vi "Turn Right.vi"() -> ()   [LabVIEW 2017]
uses:
  <vilib>/Rock Robotics/SystemInterfaces/DIO/FPGA_DIOPWMChannel.ctl
  <vilib>/Rock Robotics/SystemInterfaces/DIO/FPGA_DIOChannel.ctl
  <vilib>/Rock Robotics/WPI/MotorControl/WPI_MotorControlOpen SPARK.vi
  <vilib>/Rock Robotics/WPI/Counter/WPI_CounterDigitalInputToDigitalSource.vi
panel:
  out "Distance 2":dbl
  out "Distance":dbl
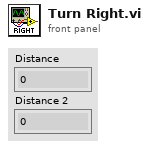
[diagram p1: front panel]
types:
  T1 = typedef "FPGA_DIOChannel.ctl" = enum8{"DIO 0", "DIO 1", "DIO 2", "DIO 3", "DIO 4", "DIO 5", "DIO 6", "DIO 7", "DIO 8", "DIO 9", "DIO MXP 0", "DIO MXP 1", "DIO MXP 2", "DIO MXP 3", "DIO MXP 4", "DIO MXP 5", "DIO MXP 6", "DIO MXP 7", "DIO MXP 8", "DIO MXP 9", "DIO MXP 10", "DIO MXP 11", "DIO MXP 12", "DIO MXP 13", "DIO MXP 14", "DIO MXP 15", "SPI Port CS1", "SPI Port CS2", "SPI Port CS3", "SPI Port MISO", "SPI Port MOSI", "Invalid"}
  T2 = typedef "FPGA_DIOPWMChannel.ctl" = enum8{"PWM 0", "PWM 1", "PWM 2", "PWM 3", "PWM 4", "PWM 5", "PWM 6", "PWM 7", "PWM 8", "PWM 9", "PWM MXP 0", "PWM MXP 1", "PWM MXP 2", "PWM MXP 3", "PWM MXP 4", "PWM MXP 5", "PWM MXP 6", "PWM MXP 7", "PWM MXP 8", "PWM MXP 9", "Invalid"}
  T3 = typedef "WPI_DigitalInputDevRef.ctl" = cluster{"DevStatus":errorcluster, "DIO Channel":T1}
  T4 = typedef "FPGA_CounterEncoderSourceConvertionLVSourceType.ctl" = cluster{"DevStatus":errorcluster, "AnalogTriggerMode?":bool, "DigitalMode":cluster{"DIO Channel":T5}, "AnalogTriggerMode":cluster{"AnalogTriggerIndex":T6, "OutputType":T7}}
  T5 = typedef "FPGA_DIODigitalSourceChannel.ctl" = enum8{"DIO 0", "DIO 1", "DIO 2", "DIO 3", "DIO 4", "DIO 5", "DIO 6", "DIO 7", "DIO 8", "DIO 9", "DIO MXP 0", "DIO MXP 1", "DIO MXP 2", "DIO MXP 3", "DIO MXP 4", "DIO MXP 5", "DIO MXP 6", "DIO MXP 7", "DIO MXP 8", "DIO MXP 9", "DIO MXP 10", "DIO MXP 11", "DIO MXP 12", "DIO MXP 13", "DIO MXP 14", "DIO MXP 15", "Disabled"}
  T6 = typedef "FPGA_AnalogTriggerIndex.ctl" = enum8{"Trig 0", "Trig 1", "Trig 2", "Trig 3", "Trig 4", "Trig 5", "Trig 6", "Trig 7", "Invalid"}
  T7 = typedef "FPGA_AnalogTriggerOutType.ctl" = enum16{"InWindow", "TriggerState", "Rising", "Falling"}
  T8 = typedef "WPI_EncoderDevRef.ctl" = cluster{"DevStatus":errorcluster, "EncoderIndex":T9, "CounterIndex":T10, "DistancePerCount":dbl, "Decoding Type":T11}
  T9 = typedef "FPGA_EncoderIdx.ctl" = enum8{"Enc 0", "Enc 1", "Enc 2", "Enc 3", "Enc 4", "Enc 5", "Enc 6", "Enc 7", "Invalid"}
  T10 = typedef "FPGA_CounterCtrSystemIndex.ctl" = enum8{"Ctr 0", "Ctr 1", "Ctr 2", "Ctr 3", "Ctr 4", "Ctr 5", "Ctr 6", "Ctr 7", "Invalid"}
  T11 = typedef "WPI_EncoderType.ctl" = enum16{"1x", "2x", "4x"}
  T12 = typedef "WPI_MotorControlDeviceRef.ctl" = cluster{"DeviceStatus":errorcluster, "Type":T13, "PWM":cluster{"PWM Channel":T2, "DeadBand":T14}, "CAN":cluster{"Device Number":u8, "SetOutput VI Ref":variant, "GetOutput VI Ref":variant, "Enable VI Ref":variant, "Disable VI Ref":variant, "Data":variant}, "Invert":bool, "DIO PWM":cluster{"PWM \"Enable\" Channel":T2, "DIOChannel":T1, "PWM Rate":dbl}}
  T13 = typedef "WPI_MotorControlType.ctl" = enum16{"PWM", "CAN", "DIO PWM"}
  T14 = typedef "WPI_PWMDeadband.ctl" = cluster{"Name":string, "maxPositivePwm":i32, "minPositivePwm":i32, "centerPwm":i32, "maxNegativePwm":i32, "minNegativePwm":i32, "angularRange":u16}
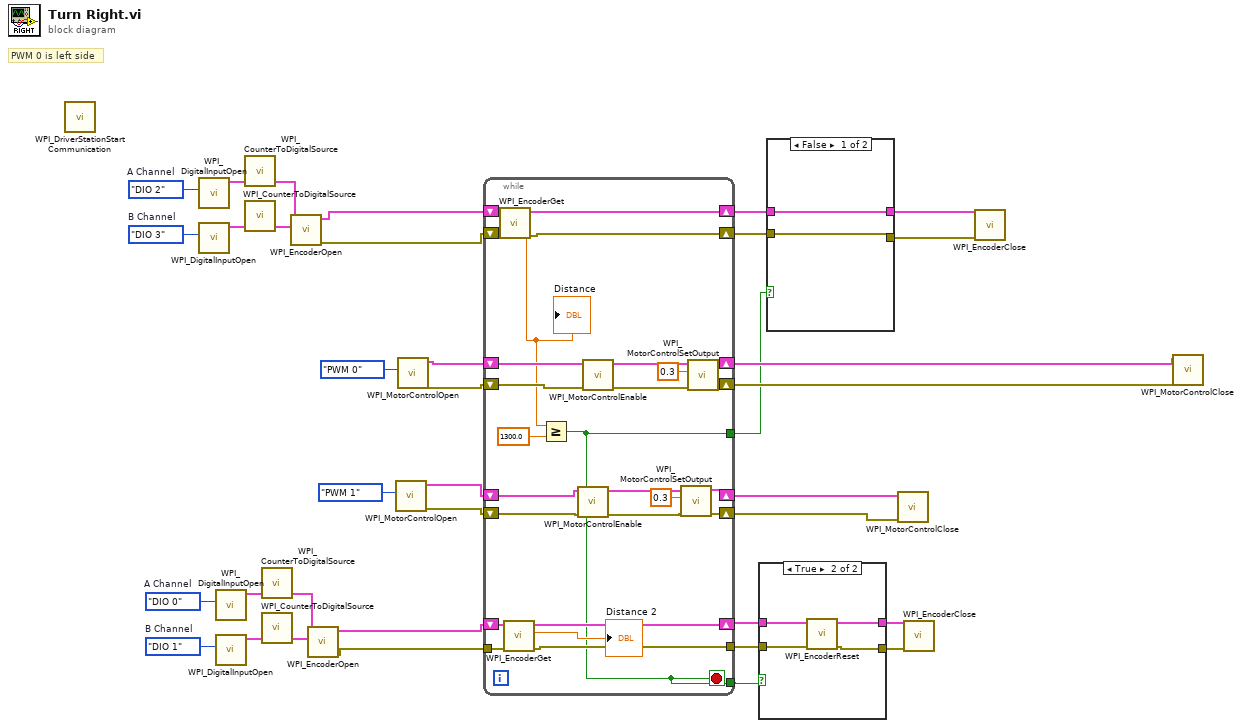
[diagram p0: block diagram]
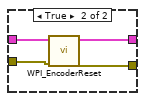
[diagram p3: hidden frame]
diagram:
  w13 = FPGA_DIOChannel."DIO 1"  # B Channel
  w14 = FPGA_DIOChannel."DIO 0"  # A Channel
  w33 = FPGA_DIOChannel."DIO 3"  # B Channel
  w32 = FPGA_DIOChannel."DIO 2"  # A Channel
  # "PWM 0 is left side"
  n1 = call <vilib>:"WPI_DriverStationStart Communication.vi"() -> ()  [unwired: 12 in]
  n2 = call <vilib>:"WPI_DigitalInputOpen.vi"("DIO Channel"=w32) -> ("DigitalInputDevRef"=w29:T3)  [unwired: 1 in, 9 out]
  n3 = call <vilib>:"WPI_DigitalInputOpen.vi"("DIO Channel"=w33) -> ("DigitalInputDevRef"=w30:T3)  [unwired: 1 in, 9 out]
  n4 = call <vilib>:"WPI_DigitalInputOpen.vi"("DIO Channel"=w14) -> ("DigitalInputDevRef"=w17:T3)  [unwired: 1 in, 9 out]
  n5 = call <vilib>:"WPI_DigitalInputOpen.vi"("DIO Channel"=w13) -> ("DigitalInputDevRef"=w16:T3)  [unwired: 1 in, 9 out]
  n6 = call-poly <vilib>:"WPI_CounterToDigitalSource.vi"("DigitalInputDevRef"=w29) -> ("Digital Source"=w28:T4)  [unwired: 6 out]
  n7 = call-poly <vilib>:"WPI_CounterToDigitalSource.vi"("DigitalInputDevRef"=w30) -> ("Digital Source"=w31:T4)  [unwired: 6 out]
  n8 = call-poly <vilib>:"WPI_CounterToDigitalSource.vi"("DigitalInputDevRef"=w17) -> ("Digital Source"=w18:T4)  [unwired: 6 out]
  n9 = call-poly <vilib>:"WPI_CounterToDigitalSource.vi"("DigitalInputDevRef"=w16) -> ("Digital Source"=w15:T4)  [unwired: 6 out]
  n10 = call <vilib>:"WPI_EncoderOpen.vi"("BSource"=w31, "ASource"=w28) -> ("error out"=w27:errorcluster, "EncoderDevRef"=w26:T8)  [unwired: 6 in, 2 out]
  n11 = call <vilib>:"WPI_EncoderOpen.vi"("BSource"=w15, "ASource"=w18) -> ("error out"=w6:errorcluster, "EncoderDevRef"=w12:T8)  [unwired: 6 in, 2 out]
  n12 = call-poly <vilib>:"WPI_MotorControlOpen.vi"("PWM Channel"=FPGA_DIOPWMChannel."PWM 1") -> ("error out"=w20:errorcluster, "MotorControlDeviceRef"=w23:T12)  [unwired: 9 in]
  n13 = call-poly <vilib>:"WPI_MotorControlOpen.vi"("PWM Channel"=FPGA_DIOPWMChannel."PWM 0") -> ("error out"=w24:errorcluster, "MotorControlDeviceRef"=w35:T12)  [unwired: 9 in]
  n14 = while {
    shift-right: [w62] -> w36
    shift-left: w35 -> [w61]
    shift-right: [w40] -> w4
    shift-left: w27 -> [w60]
    shift-right: [w41] -> w5
    shift-left: w26 -> [w59]
    shift-right: [w58] -> w25
    shift-left: w24 -> [w57]
    shift-right: [w55] -> w22
    shift-left: w23 -> [w56]
    shift-right: [w54] -> w21
    shift-left: w20 -> [w53]
    shift-right: [w51] -> w10
    shift-left: w12 -> [w52]
    tunnel: [w37] -> w11
    tunnel: [w39] -> w7
    tunnel: w6 -> [w38]
    tunnel: [w37] -> w1
    stop <- w37 stop-if-true
    n15 = call <vilib>:"WPI_EncoderGet.vi"("error in (no error)"=w60, "EncoderDevRef"=w59) -> ("error out"=w40:errorcluster, "Distance"=w43:dbl, "EncoderDevRef"=w41:T8)  [unwired: 4 in, 3 out]
    "Distance" <- w43
    n16 = call <vilib>:"WPI_EncoderGet.vi"("error in (no error)"=w38, "EncoderDevRef"=w52) -> ("error out"=w39:errorcluster, "Distance"=→"Distance 2":dbl, "EncoderDevRef"=w51:T8)  [unwired: 4 in, 3 out]
    n17 = Greater Or Equal?(x=w43, y=1300.0) -> (x >= y?=w37:bool)
    n18 = call <vilib>:"WPI_MotorControlEnable.vi"("error in (no error)"=w53, "CAN MotorDevRef"=w56) -> ("error out"=w46:errorcluster, "CAN MotorDevRef"=w47:T12)  [unwired: 8 in]
    n19 = call <vilib>:"WPI_MotorControlEnable.vi"("error in (no error)"=w57, "CAN MotorDevRef"=w61) -> ("error out"=w48:errorcluster, "CAN MotorDevRef"=w50:T12)  [unwired: 8 in]
    n20 = call <vilib>:"WPI_MotorControlSetOutput.vi"("error in (no error)"=w46, "Output"=0.3, "MotorControlDevRef"=w47) -> ("error out"=w54:errorcluster, "MotorControlDevRef"=w55:T12)  [unwired: 6 in, 1 out]
    n21 = call <vilib>:"WPI_MotorControlSetOutput.vi"("error in (no error)"=w48, "Output"=0.3, "MotorControlDevRef"=w50) -> ("error out"=w58:errorcluster, "MotorControlDevRef"=w62:T12)  [unwired: 6 in, 1 out]
  }
  n22 = case shown="True" w1 {
    tunnel: w10 -> [w64 w68]
    tunnel: [w64 w67] -> w9
    tunnel: [w63 w66] -> w8
    tunnel: w7 -> [w63 w65]
    frame False {
    }
    frame True {
      n23 = call <vilib>:"WPI_EncoderReset.vi"("error in (no error)"=w65, "EncoderDevRef"=w68) -> ("error out"=w66:errorcluster, "EncoderDevRef"=w67:T8)  [unwired: 8 in]
    }
  }
  n24 = case shown="False" w11 {
    tunnel: w5 -> [w70 w74]
    tunnel: w4 -> [w69 w73]
    tunnel: [w70 w72] -> w3
    tunnel: [w69 w71] -> w2
    frame False {
    }
    frame True {
      n25 = call <vilib>:"WPI_EncoderReset.vi"("error in (no error)"=w73, "EncoderDevRef"=w74) -> ("error out"=w71:errorcluster, "EncoderDevRef"=w72:T8)  [unwired: 8 in]
    }
  }
  n26 = call <vilib>:"WPI_MotorControlClose.vi"("error in"=w21, "MotorControlDevRef"=w22) -> ()  [unwired: 9 in, 1 out]
  n27 = call <vilib>:"WPI_EncoderClose.vi"("error in (no error)"=w8, "EncoderDevRef"=w9) -> ()  [unwired: 9 in, 1 out]
  n28 = call <vilib>:"WPI_EncoderClose.vi"("error in (no error)"=w2, "EncoderDevRef"=w3) -> ()  [unwired: 9 in, 1 out]
  n29 = call <vilib>:"WPI_MotorControlClose.vi"("error in"=w25, "MotorControlDevRef"=w36) -> ()  [unwired: 9 in, 1 out]
